vi "Cleanup Session.vi"(8 "error in":errorcluster, 11 "Plugin in":refnum<class "Adjust Block Size.lvclass">) -> (0 "error out":errorcluster, 3 "Plugin out":refnum<class "Adjust Block Size.lvclass">)   [LabVIEW 2024, in "Adjust Block Size.lvlib" / "Adjust Block Size.lvclass"]
uses:
  Adjust Block Size.lvclass
  Adjust Block Size.lvclass/Adjust Block Size.ctl
  <vilib>/addons/_NISVFA/_Shared subVIs/Data Objects/Waveforms (DBL)/Waveforms (N Ch).lvclass
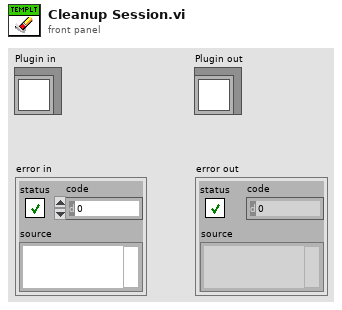
[diagram p1: front panel]
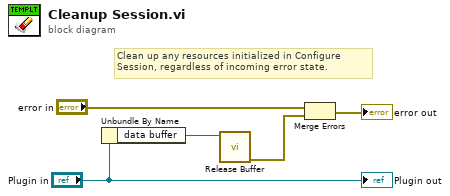
[diagram p0: block diagram]
diagram:
  # "Clean up any resources initialized in Configure Session, regardless of incoming error state."
  n1 = Unbundle By Name("Plugin in") -> ("data buffer"=w2:refnum<data-value>)
  n2 = call <vilib>:"Release Buffer.vi"("buffer"=w2) -> ("error out"=w1:errorcluster)  [unwired: 10 in]
  n3 = Merge Errors("error in", w1) -> (→"error out":errorcluster)
  "Plugin out" <- "Plugin in"
